vi "SENS_FREQ_STOP.vi"(0 "VISA IN":refnum<visa-resource-name>, 1 "Frq. Stop":dbl, 5 "error in":errorcluster, 7 "Channel":i32=1) -> (14 "VISA Out":refnum<visa-resource-name>, 19 "error out":errorcluster)   [LabVIEW 2018, in "PNA-X.lvlib"]
doc: "SENSe<cnum>:FREQuency:STOP <num> \n(Read-Write) Sets the stop frequency of the analyzer. \nParameters \n<cnum> Any existing channel number. If unspecified, value is set to 1 \n<num> Stop frequency. Choose any number between: \nthe minimum and maximum frequency limits of the analyzer. Units are Hz \nIf FREQ:STOP is set less than FREQ:START, then START will be set equal to \nSTOP. \nSee Note \nExamples SENS:FREQ:STOP 1000000 \nsense2:frequency:stop max \nQuery Syntax SENSe<cnum>:FREQuency:STOP? \nIf Sweep type is segment, this query returns the stop frequency of the last segment. \nReturn Type Numeric \nDefault Maximum frequency of the analyzer \n1746\n\n1747\n\nSense:IF Commands \nControls the IF source and gain settings for use with the E836x H11 Option. \nSee IF/DSP and Pulse commands for the PNA-X. \nClick on a blue keyword to view the command details. \nSee IF Access User Interface Settings \nSynchronizing the PNA and Controller \nSCPI Command Tree"
uses:
  PNA-X.lvlib
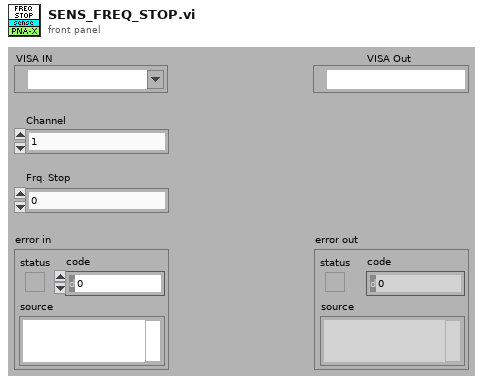
[diagram p1: front panel]
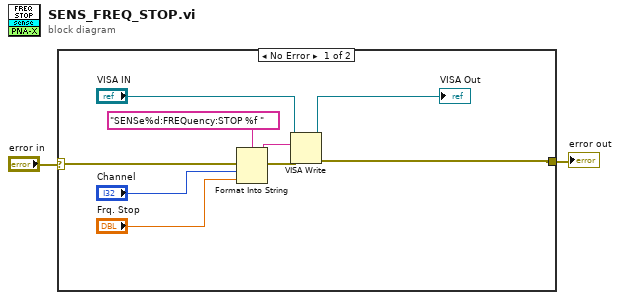
[diagram p0: block diagram]
diagram:
  n1 = case shown="No Error" "error in" {
    selector: "error in" -> [w11 w12]
    tunnel: [w6 w12] -> w1
    frame No Error {
      n2 = Format Into String(format string="SENSe%d:FREQuency:STOP %f " ("Cmdline"), error in=w11, "Channel", "Frq. Stop") -> (resulting string=w9:string, error out=w10:errorcluster)  [unwired: 1 in]
      n3 = VISA Write(VISA resource name="VISA IN", write buffer=w9, error in (no error)=w10) -> (VISA resource name out=→"VISA Out":refnum<visa-resource-name>, error out=w6:errorcluster)  [unwired: 1 out]
    }
    frame Error {
    }
  }
  "error out" <- w1
